vi "SaveHands.vi"(10 "error in (no error)":errorcluster, 11 ".NET Refnum in":refnum<k24>) -> (2 "error out":errorcluster, 3 "Hands":T1[](array[typedef]))   [LabVIEW 2011, in "LVH-Leap.lvlib"]
uses:
  LVH-Leap.lvlib
  Type Defs/Hand.ctl
  Type Defs/Vector.ctl
  Type Defs/Pointable.ctl
  Type Defs/Pointable Type.ctl
  Type Defs/Pointable Zone.ctl
  C:/github/labviewhacker/LVH-Leap/LabVIEW/vi.lib/LabVIEW Hacker/Leap/Private/Libs/LeapCSharp.NET3.5.dll
  Libs/LeapCSharp.NET3.5.dll
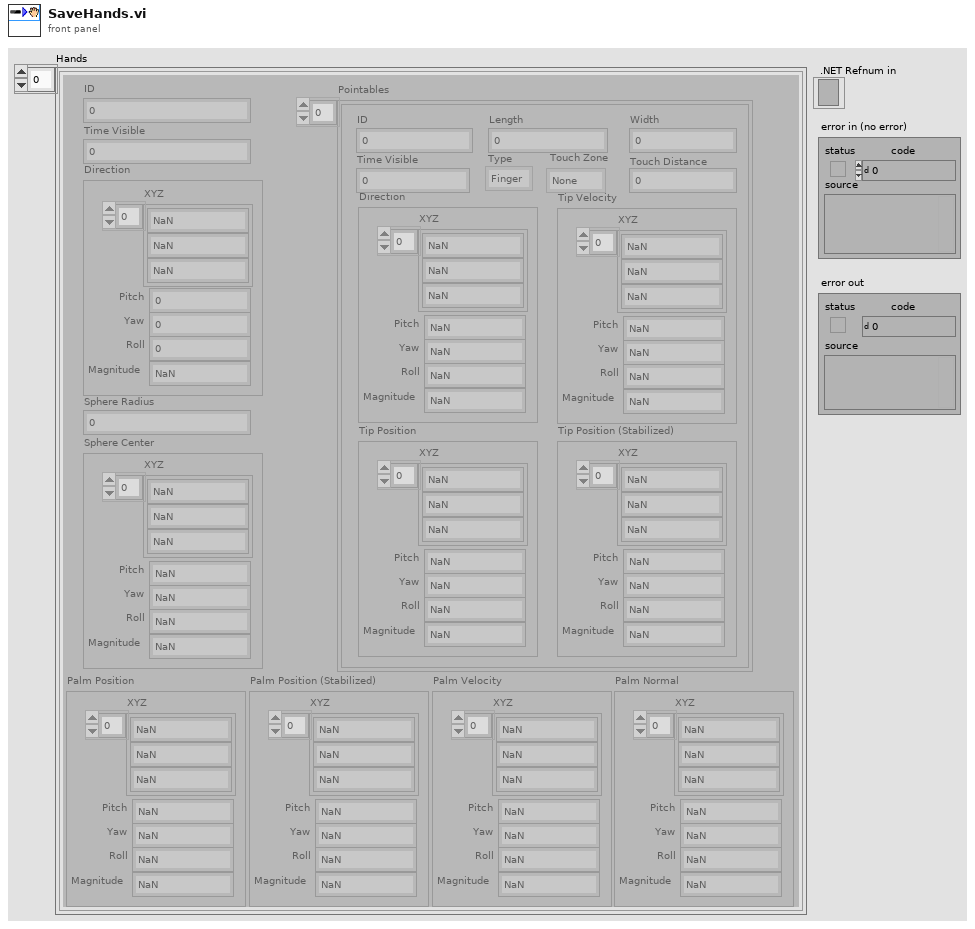
[diagram p1: front panel]
types:
  T1 = typedef "LVH-Leap.lvlib/Hand.ctl" = cluster{"ID":i32, "Time Visible":sgl, "Direction":T2, "Palm Position":T2, "Palm Position (Stabilized)":T2, "Palm Velocity":T2, "Palm Normal":T2, "Pointables":T3[], "Sphere Radius":sgl, "Sphere Center":T2}
  T2 = typedef "LVH-Leap.lvlib/Vector.ctl" = cluster{"Pitch":sgl, "Yaw":sgl, "Roll":sgl, "Magnitude":sgl, "XYZ":sgl[]}
  T3 = typedef "LVH-Leap.lvlib/Pointable.ctl" = cluster{"ID":i32, "Length":dbl, "Width":dbl, "Time Visible":dbl, "Type":T4, "Direction":T2, "Tip Velocity":T2, "Tip Position":T2, "Tip Position (Stabilized)":T2, "Touch Zone":T5, "Touch Distance":dbl}
  T4 = typedef "LVH-Leap.lvlib/Pointable Type.ctl" = enum16{"Finger", "Tool"}
  T5 = typedef "LVH-Leap.lvlib/Pointable Zone.ctl" = enum16{"None", "Hovering", "Touching"}
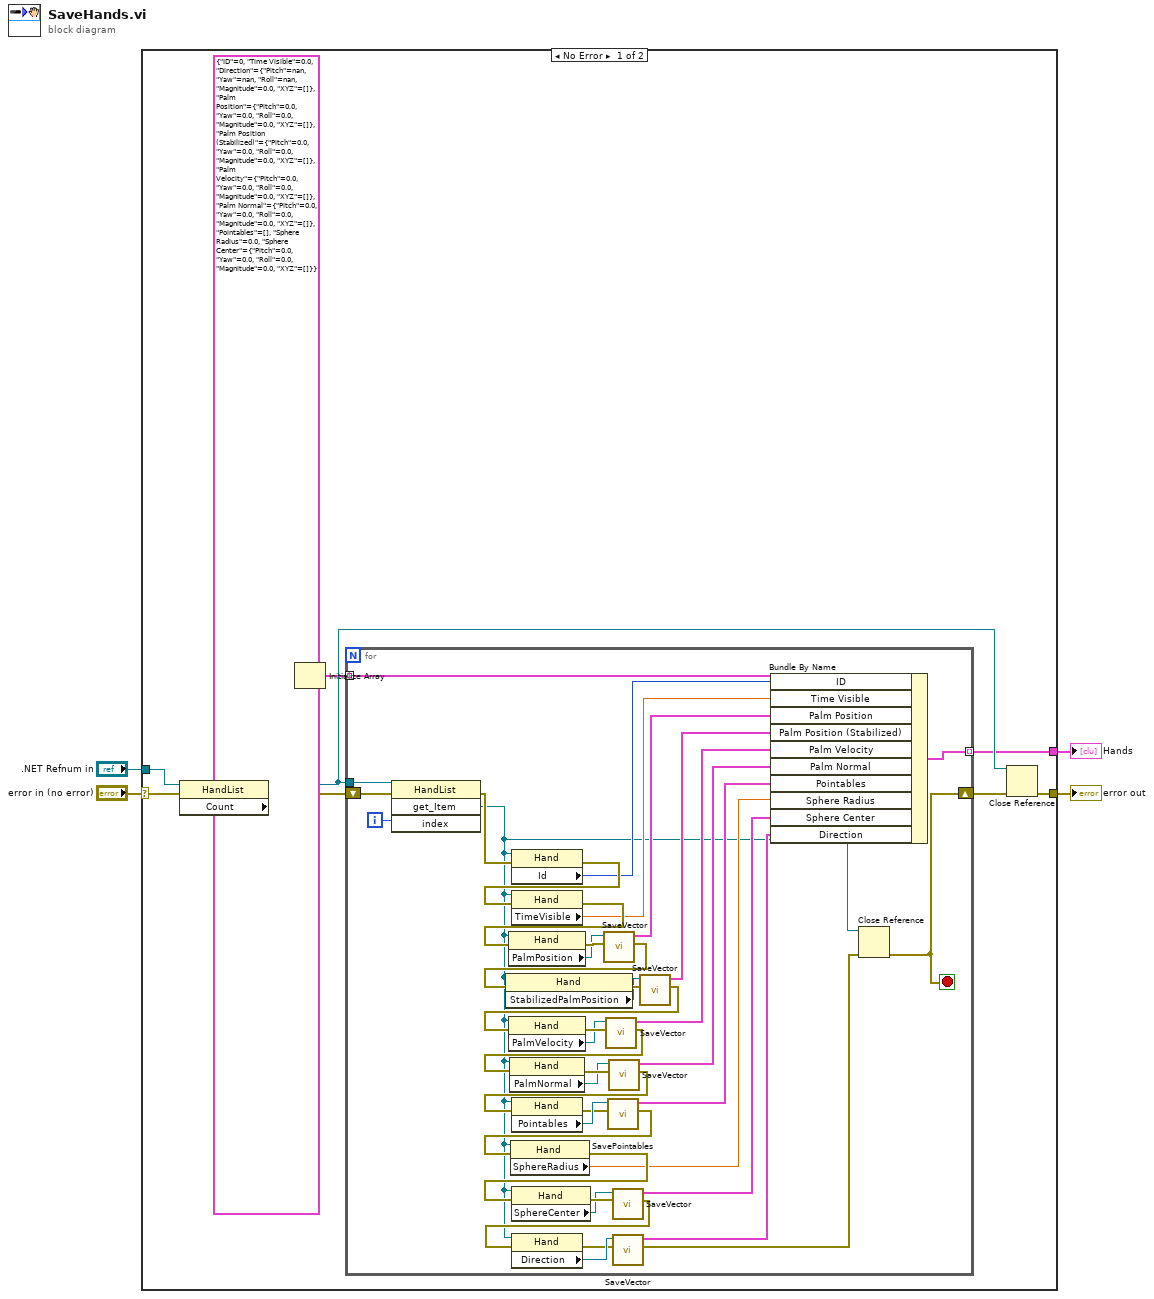
[diagram p0: block diagram]
diagram:
  n1 = case shown="No Error" "error in (no error)" {
    selector: "error in (no error)" -> [w7 w57]
    tunnel: [w12 _] -> w4
    tunnel: ".NET Refnum in" -> [w8 _]
    tunnel: [w5 w57] -> w2
    frame No Error {
      n2 = property class="HandList"(reference=w8, error in=w7) -> (reference out=w13:refnum<k24>, error out=w14:errorcluster, "Count"=w9:i32)
      n3 = Initialize Array(T1 {"ID"=0, "Time Visible"=0.0, "Direction"={"Pitch"=nan, "Yaw"=nan, "Roll"=nan, "Magnitude"=0.0, "XYZ"=[]}, "Palm Position"={"Pitch"=0.0, "Yaw"=0.0, "Roll"=0.0, "Magnitude"=0.0, "XYZ"=[]}, "Palm Position (Stabilized)"={"Pitch"=0.0, "Yaw"=0.0, "Roll"=0.0, "Magnitude"=0.0, "XYZ"=[]}, "Palm Velocity"={"Pitch"=0.0, "Yaw"=0.0, "Roll"=0.0, "Magnitude"=0.0, "XYZ"=[]}, "Palm Normal"={"Pitch"=0.0, "Yaw"=0.0, "Roll"=0.0, "Magnitude"=0.0, "XYZ"=[]}, "Pointables"=[], "Sphere Radius"=0.0, "Sphere Center"={"Pitch"=0.0, "Yaw"=0.0, "Roll"=0.0, "Magnitude"=0.0, "XYZ"=[]}} ("Hand"), w9) -> (w11:T1[])
      n4 = for {
        tunnel: w13 -> [w43]
        tunnel: w11 -> [w41] mode=indexing
        tunnel: [w39] -> w12 mode=indexing
        shift-right: [w33] -> w6
        shift-left: w14 -> [w44]
        i -> [w42]
        stop <- w33 stop-if-true
        n5 = invoke class="HandList" method="get_Item"(reference=w43, error in=w44, "index"=w42) -> (error out=w51:errorcluster, "get_Item"=w15:refnum<k24>)  [unwired: 1 in, 2 out]
        n6 = property class="Hand"(reference=w15, error in=w51) -> (error out=w50:errorcluster, "Id"=w40:i32)  [unwired: 1 out]
        n7 = property class="Hand"(reference=w15, error in=w50) -> (error out=w47:errorcluster, "TimeVisible"=w32:sgl)  [unwired: 1 out]
        n8 = property class="Hand"(reference=w15, error in=w47) -> (error out=w31:errorcluster, "PalmPosition"=w30:refnum<k24>)  [unwired: 1 out]
        n9 = call "SaveVector.vi"("error in (no error)"=w31, "Leap Vector"=w30) -> ("error out"=w49:errorcluster, "Vector"=w28:T2)  [unwired: 8 in]
        n10 = property class="Hand"(reference=w15, error in=w49) -> (error out=w45:errorcluster, "StabilizedPalmPosition"=w29:refnum<k24>)  [unwired: 1 out]
        n11 = call "SaveVector.vi"("error in (no error)"=w45, "Leap Vector"=w29) -> ("error out"=w52:errorcluster, "Vector"=w27:T2)  [unwired: 8 in]
        n12 = property class="Hand"(reference=w15, error in=w52) -> (error out=w46:errorcluster, "PalmVelocity"=w38:refnum<k24>)  [unwired: 1 out]
        n13 = call "SaveVector.vi"("error in (no error)"=w46, "Leap Vector"=w38) -> ("error out"=w53:errorcluster, "Vector"=w26:T2)  [unwired: 8 in]
        n14 = property class="Hand"(reference=w15, error in=w53) -> (error out=w37:errorcluster, "PalmNormal"=w36:refnum<k24>)  [unwired: 1 out]
        n15 = call "SaveVector.vi"("error in (no error)"=w37, "Leap Vector"=w36) -> ("error out"=w54:errorcluster, "Vector"=w25:T2)  [unwired: 8 in]
        n16 = property class="Hand"(reference=w15, error in=w54) -> (error out=w23:errorcluster, "Pointables"=w24:refnum<k24>)  [unwired: 1 out]
        n17 = call "SavePointables.vi"("error in (no error)"=w23, "Leap Pointables"=w24) -> ("error out"=w48:errorcluster, "Pointables"=w22:T3[])  [unwired: 8 in]
        n18 = property class="Hand"(reference=w15, error in=w48) -> (error out=w55:errorcluster, "SphereRadius"=w21:sgl)  [unwired: 1 out]
        n19 = property class="Hand"(reference=w15, error in=w55) -> (error out=w35:errorcluster, "SphereCenter"=w34:refnum<k24>)  [unwired: 1 out]
        n20 = call "SaveVector.vi"("error in (no error)"=w35, "Leap Vector"=w34) -> ("error out"=w16:errorcluster, "Vector"=w20:T2)  [unwired: 8 in]
        n21 = property class="Hand"(reference=w15, error in=w16) -> (error out=w18:errorcluster, "Direction"=w19:refnum<k24>)  [unwired: 1 out]
        n22 = call "SaveVector.vi"("error in (no error)"=w18, "Leap Vector"=w19) -> ("error out"=w17:errorcluster, "Vector"=w56:T2)  [unwired: 8 in]
        n23 = Bundle By Name(cluster=w41, "ID"=w40, "Time Visible"=w32, "Palm Position"=w28, "Palm Position (Stabilized)"=w27, "Palm Velocity"=w26, "Palm Normal"=w25, "Pointables"=w22, "Sphere Radius"=w21, "Sphere Center"=w20, "Direction"=w56) -> (w39:T1)
        n24 = Close Reference(reference=w15, error in (no error)=w17) -> (error out=w33:errorcluster)
      }
      n25 = Close Reference(reference=w13, error in (no error)=w6) -> (error out=w5:errorcluster)
    }
    frame Error {
    }
  }
  "Hands" <- w4
  "error out" <- w2
